vi "Global.Salir Ya.vi"() -> ()   [LabVIEW 2019]
panel:
  in  "Cancel":bool
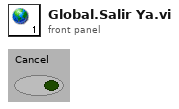
[diagram p1: front panel]
diagram:
